vi "U Boat main.vi"() -> ()   [LabVIEW 2013]
uses:
  <vilib>/Utility/inputDevices.llb/closeJoystick.vi
  <vilib>/Utility/inputDevices.llb/joystickAcquire.vi
panel:
  in  "VISA resource name":refnum<visa-resource-name>="COM7"
  out "XBee ?":bool
  in  "String":string="$CS1500L1\n"
  out "bytes written":u32
  out "return count":u32
  out "String Received":string
  in  "Rudder\nOffset":i16(slide) min=-100 max=100 step=1 scale=-100.0..100.0
  out "Jib Sheet":u16=1500
  out "Main sheet":u16=1500
  out "Rudder":u16=1500
  out "error out":errorcluster
  in  "stop":bool
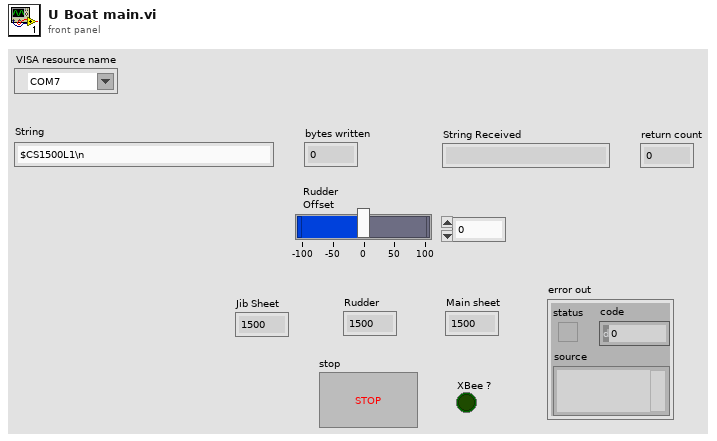
[diagram p1: front panel]
types:
  T1 = cluster{"X axis":i32, "Y axis":i32, "Z axis":i32, "X axis rotation":i32, "Y axis rotation":i32, "Z axis rotation":i32, "U axis":i32, "V axis":i32}
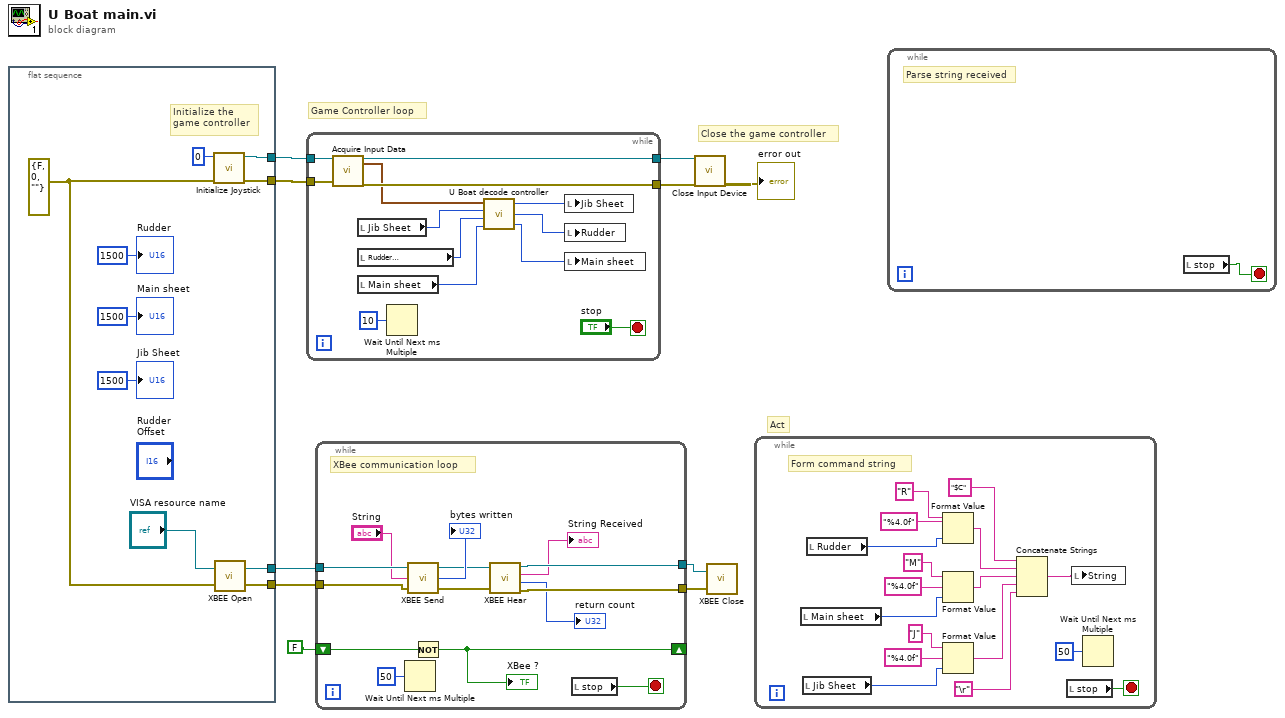
[diagram p0: block diagram]
diagram:
  # "Act"
  # "Close the game controller"
  # "Game Controller loop"
  n1 = flat-sequence {
    tunnel: [w19] -> w10
    tunnel: [w18] -> w8
    tunnel: [w16] -> w3
    tunnel: [w15] -> w2
    frame #0 {
      w11 = errorcluster {"status"=FALSE, "code"=0, "source"=""} ("error in (no error)")
      # "Initialize the\ngame controller"
      n2 = call <vilib>:"Initialize Joystick.vi"("error in (no error)"=w11, "device index"=0) -> ("error out"=w18:errorcluster, "device ID"=w19:refnum<k1>)  [unwired: 8 in]
      n3 = call "XBEE Open.vi"("error in"=w11, "VISA resource name"="VISA resource name") -> ("error out"=w15:errorcluster, "VISA resource name out"=w16:refnum<visa-resource-name>)
      "Rudder" <- u16 1500 ("MRudder")
      "Main sheet" <- u16 1500 ("MRudder")
      "Jib Sheet" <- u16 1500 ("MRudder")
    }
  }
  n4 = while {
    tunnel: w10 -> [w33]
    tunnel: [w32] -> w9
    tunnel: w8 -> [w31]
    tunnel: [w30] -> w7
    stop <- "stop" stop-if-true
    n5 = call-poly <vilib>:"Acquire Input Data.vi"("device ID"=w33, "error in (no error)"=w31) -> ("device ID"=w32:refnum<k1>, "axis info"=w27:T1, "error out"=w30:errorcluster)  [unwired: 13 in, 2 out]
    n6 = local read "Jib Sheet"() -> (w26:u16)
    n7 = local read "Rudder\nOffset"() -> (w21:i16)
    n8 = local read "Main sheet"() -> (w25:u16)
    n9 = Wait Until Next ms Multiple(millisecond multiple=u32 10) -> ()  [unwired: 1 out]
    n10 = call "U Boat decode controller.vi"("Main sheet In"=w25, "Rudder\nOffset"=w21, "Jib Sheet In"=w26, "axis info"=w27) -> ("Main sheet Out"=w23:u16, "Rudder Out"=w24:u16, "Jib Steet Out"=w22:u16)
    n11 = local write "Jib Sheet"(w22) -> ()
    n12 = local write "Rudder"(w24) -> ()
    n13 = local write "Main sheet"(w23) -> ()
  }
  n14 = while {
    tunnel: w3 -> [w47]
    tunnel: w2 -> [w46]
    tunnel: [w41] -> w5
    tunnel: [w40] -> w4
    shift-right: [w44] -> _
    shift-left: FALSE -> [w45]
    stop <- w34 stop-if-true
    # "XBee communication loop"
    n15 = Wait Until Next ms Multiple(millisecond multiple=u32 50) -> ()  [unwired: 1 out]
    n16 = call "XBEE Send.vi"("error in (no error)"=w46, "String"="String", "VISA resource name"=w47) -> ("error out"=w37:errorcluster, "return count"=→"bytes written":u32, "VISA resource name out"=w38:refnum<visa-resource-name>)
    n17 = Not(x=w45) -> (.not. x?=w44:bool)
    "XBee ?" <- w44
    n18 = call "XBEE Hear.vi"("VISA resource name"=w38, "error in (no error)"=w37) -> ("VISA resource name out"=w41:refnum<visa-resource-name>, "String Received"=→"String Received":string, "return count"=→"return count":u32, "error out"=w40:errorcluster)
    n19 = local read "stop"() -> (w34:bool)
  }
  n20 = call-poly <vilib>:"Close Input Device.vi"("error in (no error)"=w7, "device ID"=w9) -> ("error out"=→"error out":errorcluster)  [unwired: 8 in]
  n21 = call "XBEE Close.vi"("error in (no error)"=w4, "VISA resource name"=w5) -> ()
  n22 = while {
    stop <- w64 stop-if-true
    # "Form command string"
    n23 = local read "Main sheet"() -> (w54:u16)
    n24 = local read "Jib Sheet"() -> (w51:u16)
    n25 = local read "Rudder"() -> (w61:u16)
    n26 = Format Value(string ("")="R", format string="%4.0f", value (0)=w61) -> (output string=w59:string)
    n27 = Format Value(string ("")="M", format string="%4.0f", value (0)=w54) -> (output string=w50:string)
    n28 = Format Value(string ("")="J", format string="%4.0f", value (0)=w51) -> (output string=w49:string)
    n29 = Concatenate Strings("$C", w59, w50, w49, "\r") -> (w57:string)
    n30 = local read "stop"() -> (w64:bool)
    n31 = local write "String"(w57) -> ()
    n32 = Wait Until Next ms Multiple(millisecond multiple=u32 50) -> ()  [unwired: 1 out]
  }
  n33 = while {
    stop <- w65 stop-if-true
    # "Parse string received"
    n34 = local read "stop"() -> (w65:bool)
  }
